vi "zad2.vi"() -> ()   [LabVIEW 2025]
panel:
  out "Valid?":bool
  in  "password":string
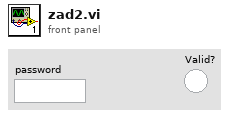
[diagram p1: front panel]
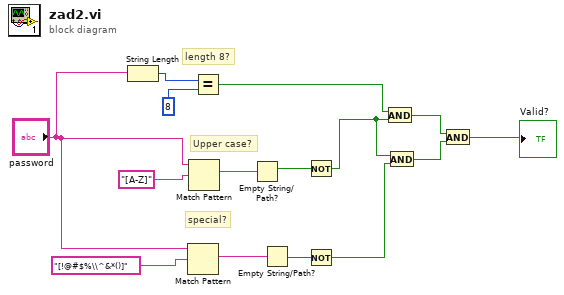
[diagram p0: block diagram]
diagram:
  # "special?"
  # "Upper case?"
  # "length 8?"
  n1 = String Length(string="password") -> (length=w15:i32)
  n2 = Match Pattern(string="password", regular expression="[!@#$%\\^&*()]") -> (match substring=w9:string)  [unwired: 1 in, 3 out]
  n3 = Match Pattern(string="password", regular expression="[A-Z]") -> (match substring=w10:string)  [unwired: 1 in, 3 out]
  n4 = Equal?(x=w15, y=8) -> (x = y?=w6:bool)
  n5 = Empty String/Path?(string/path=w10) -> (empty?=w8:bool)
  n6 = Empty String/Path?(string/path=w9) -> (empty?=w7:bool)
  n7 = Not(x=w8) -> (.not. x?=w5:bool)
  n8 = Not(x=w7) -> (.not. x?=w4:bool)
  n9 = And(x=w6, y=w5) -> (x .and. y?=w3:bool)
  n10 = And(x=w5, y=w4) -> (x .and. y?=w2:bool)
  n11 = And(x=w3, y=w2) -> (x .and. y?=→"Valid?":bool)
